vi "test Print Object Type Base.vi"(11 "Test Case In":refnum<class "test EDS.lvclass">) -> (0 "error out":errorcluster, 3 "Test Case Out":refnum<class "test EDS.lvclass">)   [LabVIEW 2024, in "test EDS.lvclass"]
uses:
  test EDS.lvclass
  C:/Program Files/National Instruments/LabVIEW 2024/vi.lib/Astemes/LUnit/Test Case.lvclass
  Core/VAR/VAR.lvclass
  <vilib>/Astemes/LUnit/Test Case.lvclass/Test Case.ctl
  e7378de1-53b1-457d-8a33-8d2c72fa2c9e.vi
  <vilib>/Astemes/LUnit/Append Pass Result.vi
  <vilib>/Astemes/LUnit/Append Fail Result.vi
  <vilib>/Astemes/LUnit/Describe Comparison.vi
  e7378de1-53b1-457d-8a33-8d2c72fa2c9e.vi/9c5d11cd-9439-4240-a1ee-d9baace9c924.vi
  <vilib>/Astemes/LUnit/Run In UI.vi
  <vilib>/Utility/error.llb/Clear Errors.vi
  <vilib>/Astemes/LUnit/Describe Variant.vi
  Core/Keyname/Key Name.lvclass
  Core/Value/Value.lvclass
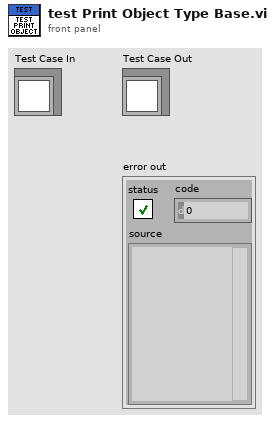
[diagram p1: front panel]
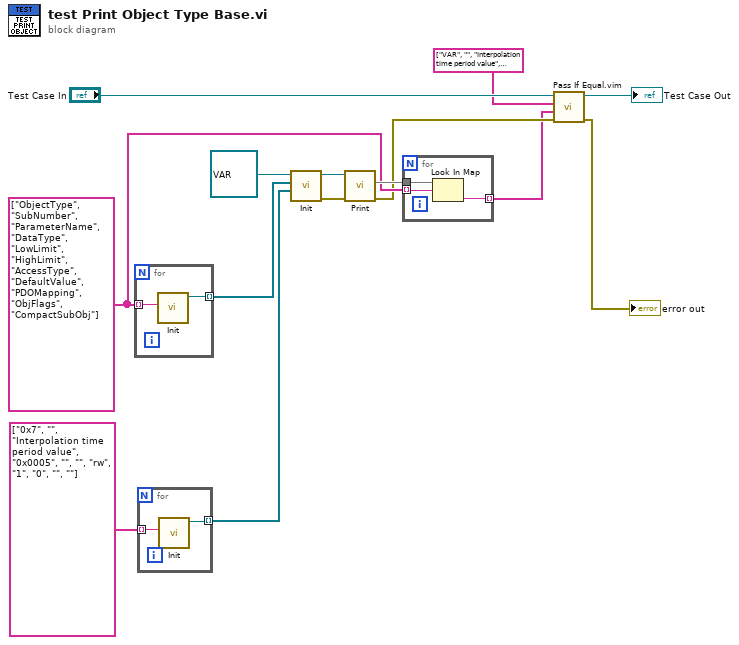
[diagram p0: block diagram]
diagram:
  w6 = string[] ["ObjectType", "SubNumber", "ParameterName", "DataType", "LowLimit", "HighLimit", "AccessType", "DefaultValue", "PDOMapping", "ObjFlags", "CompactSubObj"]
  n1 = for {
    tunnel: w6 -> [w16] mode=indexing
    tunnel: [w15] -> w10 mode=indexing
    n2 = call "Init.vi"("Key Name"=w16) -> ("Key Name out"=w15:refnum<class "Key Name.lvclass">)  [unwired: 9 in, 1 out]
  }
  n3 = for {
    tunnel: string[] ["0x7", "", "Interpolation time period value", "0x0005", "", "", "rw", "1", "0", "", ""] -> [w18] mode=indexing
    tunnel: [w17] -> w11 mode=indexing
    n4 = call "Init.vi"("Value"=w18) -> ("Value out"=w17:refnum<class "Value.lvclass">)  [unwired: 9 in, 1 out]
  }
  n5 = call-dynamic "Init.vi"("Values"=w11, "Keys"=w10, "VAR in"=refnum<class "VAR.lvclass"> refnum ("EDS.lvlib:VAR.lvclass")) -> ("error out"=w8:errorcluster, "VAR out"=w9:refnum<class "VAR.lvclass">)  [unwired: 7 in]
  n6 = call-dynamic "Print.vi"("error in"=w8, "Object Type Base in"=w9) -> ("error out"=w4:errorcluster, "Fields"=w7:map{string, string})  [unwired: 7 in, 1 out]
  n7 = for {
    tunnel: w7 -> [w21]
    tunnel: w6 -> [w20] mode=indexing
    tunnel: [w19] -> w2 mode=indexing
    n8 = Look In Map(map=w21, key=w20) -> (value=w19:string)  [unwired: 1 in, 1 out]
  }
  n9 = call "Pass If Equal.vim"("error in (no error)"=w4, "Actual"=w2, "Expected"=string[] ["VAR", "", "Interpolation time period value", "UNSIGNED8", "", "", "rw", "1", "0", "0", "0"] ("Array"), "LUnit Test Case In"="Test Case In") -> ("error out"=→"error out":errorcluster, "LUnit Test Case Out"=→"Test Case Out":refnum<class "test EDS.lvclass">)  [unwired: 6 in]
